vi "re_create_new_collection.vi"(0 "abstract_vector_base in":refnum<class "abstract_vector_base.lvclass">, 5 "collection_name":string, 7 "vector_size":u32=300, 9 "distance":string="cosine", 11 "error in (no error)":errorcluster) -> (4 "abstract_vector_base out":refnum<class "abstract_vector_base.lvclass">, 15 "error out":errorcluster)   [LabVIEW 2020, in "abstract_vector_base.lvclass"]
uses:
  abstract_vector_base.lvclass
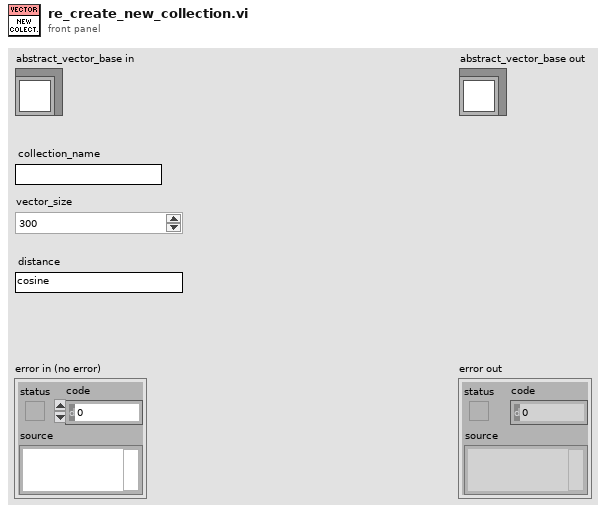
[diagram p1: front panel]
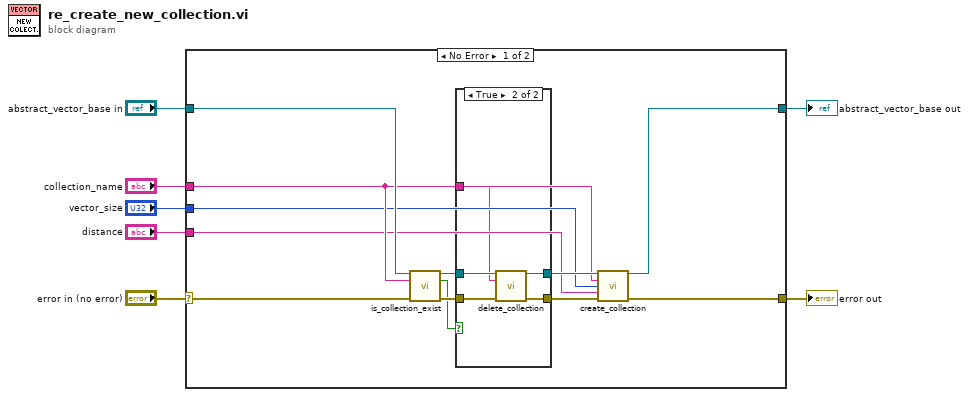
[diagram p0: block diagram]
diagram:
  n1 = case shown="No Error" "error in (no error)" {
    selector: "error in (no error)" -> [w18 w28]
    tunnel: [w10 w28] -> w6
    tunnel: [w9 w27] -> w4
    tunnel: "abstract_vector_base in" -> [w19 w27]
    tunnel: "collection_name" -> [w13 _]
    tunnel: "vector_size" -> [w12 _]
    tunnel: "distance" -> [w11 _]
    frame No Error {
      n2 = call-dynamic "is_collection_exist.vi"("abstract_vector_base in"=w19, "collection_name"=w13, "error in (no error)"=w18) -> ("abstract_vector_base out"=w16:refnum<class "abstract_vector_base.lvclass">, "exist? (True: Exist)"=w8:bool, "error out"=w17:errorcluster)  [unwired: 10 in]
      n3 = case shown="True" w8 {
        tunnel: w17 -> [w21 w26]
        tunnel: w16 -> [w20 w25]
        tunnel: [w21 w24] -> w15
        tunnel: [w20 w23] -> w14
        tunnel: w13 -> [_ w22]
        frame False {
        }
        frame True {
          n4 = call-dynamic "delete_collection.vi"("abstract_vector_base in"=w25, "collection_name"=w22, "error in (no error)"=w26) -> ("abstract_vector_base out"=w23:refnum<class "abstract_vector_base.lvclass">, "error out"=w24:errorcluster)  [unwired: 11 in]
        }
      }
      n5 = call-dynamic "create_collection.vi"("abstract_vector_base in"=w14, "collection_name"=w13, "vector_size"=w12, "distance"=w11, "error in (no error)"=w15) -> ("abstract_vector_base out"=w9:refnum<class "abstract_vector_base.lvclass">, "error out"=w10:errorcluster)  [unwired: 9 in]
    }
    frame Error {
    }
  }
  "error out" <- w6
  "abstract_vector_base out" <- w4
